vi "haoFPGA.vi"() -> ()   [LabVIEW 2018]
uses:
  <vilib>/Platform/TimedLoop/XDataNode/timing_clust.ctl
  <vilib>/Platform/TimedLoop/XDataNode/nitl_modes.ctl
  <vilib>/Platform/TimedLoop/XDataNode/wakeup.ctl
  <vilib>/rvi/Emulation/niFpgaSctlEmulationGetInTimedLoop.vi
  <vilib>/rvi/Emulation/niFpgaEmulationReportErrorSimple.vi
  <vilib>/rvi/Emulation/niFpgaGetClockAttributes.vi
  <vilib>/rvi/Emulation/niFpgaCriticalErrorInLSC.vi
  <vilib>/rvi/Emulation/niFpgaProcessEmulError.vi
  <vilib>/Platform/TimedLoop/XDataNode/XDataNode.xnode
  <vilib>/Platform/TimedLoop/XDataNode/XDNodeRunTimeDep.lvlib
panel:
  in  "B":bool
  in  "A":bool
  out "C":bool
  in  "stop":bool
  in  "DIR2":bool
  in  "ENA2":bool
  in  "STBY2":bool
  in  "CH2 DC":fxp<+,32,0>
  in  "CH1 DC":fxp<+,32,0>
  in  "STBY1":bool
  in  "ENA1":bool
  in  "DIR1":bool
  # "Motor control"
  # "Channel 1"
  # "Channel 2"
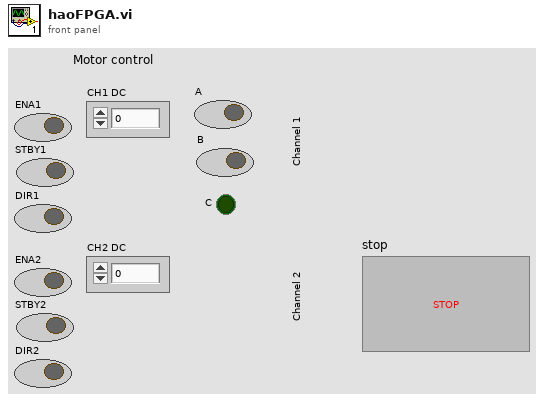
[diagram p1: front panel]
types:
  T1 = cluster{"FPGA I/O":refnum<k21>, "FPGA I/O 2":refnum<k21>, "FPGA I/O 3":refnum<k21>, "FPGA I/O 4":refnum<k21>, "FPGA I/O 5":refnum<k21>, "FPGA I/O 6":refnum<k21>, "FPGA I/O 7":refnum<k21>}
  T2 = typedef "XDNodeRunTimeDep.lvlib/timing_clust.ctl" = cluster{"Expected End [f-1]":u64, "Actual End [f-1]":u64, "Finished Late? [f-1]":bool, "Expected End [i-1]":u64, "Actual End [i-1]":u64, "Finished Late? [i-1]":bool, "Expected Start [i]":u64, "Actual Start [i]":u64, "Expected Start [f]":u64, "Actual Start [f]":u64, "Source Name":string, "Structure Name":string, "Period":i64, "Deadline":i64, "Offset":i64, "Start":i64, "Priority":i32, "Timeout":i32, "Mode":T3, "Wakeup Reason":T4, "Error":errorcluster, "Source Type":string, "Secondary Source Type":string, "Global End Time":u64, "Global Start Time":u64, "Frame Duration":u64, "Iteration Duration":u64, "Assigned CPU":i32, "I/O Scan Engine Mode":u32}
  T3 = typedef "XDNodeRunTimeDep.lvlib/nitl_modes.ctl" = enum32{"No Change", "Process missed periods, maintain original phase", "Discard missed periods, maintain original phase", "Process missed periods, ignore original phase", "Discard missed periods, ignore original phase"}
  T4 = typedef "XDNodeRunTimeDep.lvlib/wakeup.ctl" = enum32{"Normal", "Aborted", "Asynchronous wakeup", "Timing source error", "Timed loop error", "Timeout"}
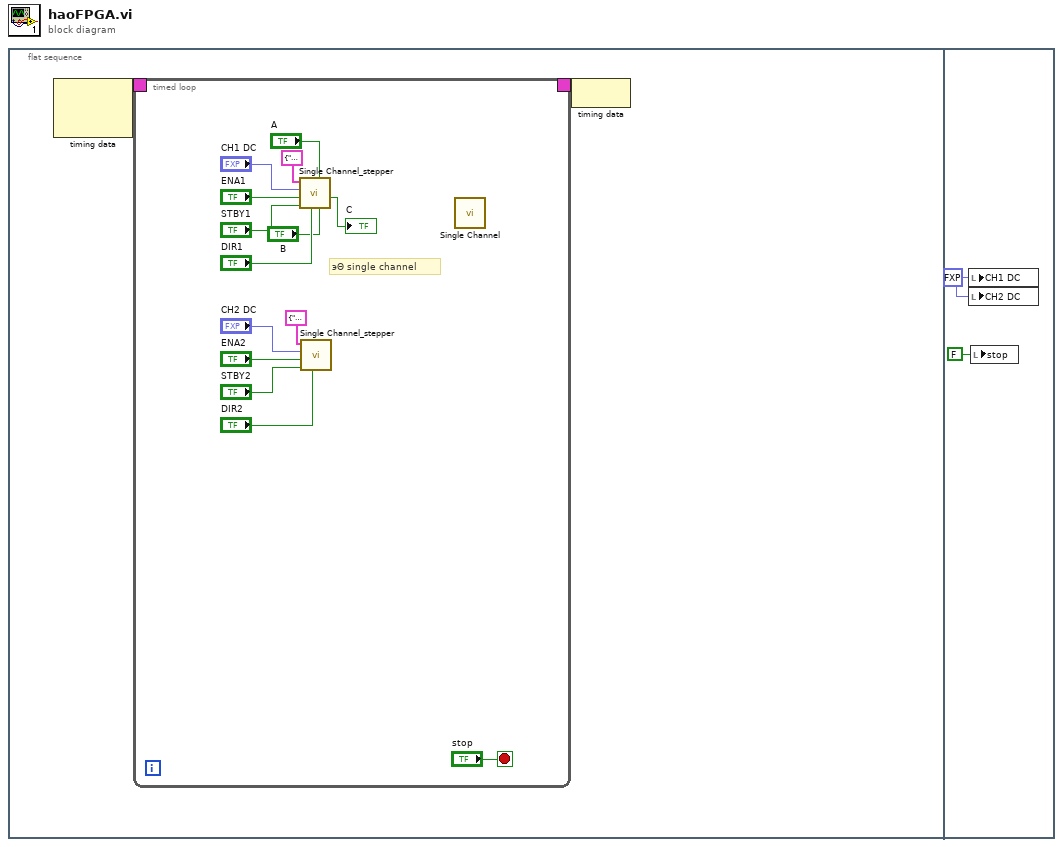
[diagram p0: block diagram]
diagram:
  n1 = flat-sequence {
    frame #0 {
      n2 = node-c288() -> (w2:T2)  [unwired: 2 in]
      n3 = timed-loop {
        timing: w2 -> [_]
        timing-out: [_] -> w1
        stop <- "stop" stop-if-true
        # "эΘ single channel"
        n4 = call "Single Channel_stepper.vi"("B"="B", "A"="A", "DIR"="DIR1", "STBY"="STBY1", "ENA"="ENA1", "Duty"="CH1 DC", "I/O Channel"=T1 {"FPGA I/O"="ConnectorA/DIO6", "FPGA I/O 2"="ConnectorA/DIO5", "FPGA I/O 3"="ConnectorA/DIO4", "FPGA I/O 4"="ConnectorA/DIO3", "FPGA I/O 5"="ConnectorA/DIO2", "FPGA I/O 6"="ConnectorA/DIO1", "FPGA I/O 7"="ConnectorA/DIO0"}) -> ("C"=→"C":bool)  [unwired: 4 in]
        n5 = call "Single Channel_stepper.vi"("DIR"="DIR2", "STBY"="STBY2", "ENA"="ENA2", "Duty"="CH2 DC", "I/O Channel"=T1 {"FPGA I/O"="ConnectorA/DIO13", "FPGA I/O 2"="ConnectorA/DIO12", "FPGA I/O 3"="ConnectorA/DIO11", "FPGA I/O 4"="ConnectorA/DIO10", "FPGA I/O 5"="ConnectorA/DIO9", "FPGA I/O 6"="ConnectorA/DIO8", "FPGA I/O 7"="ConnectorA/DIO7"}) -> ()  [unwired: 6 in, 1 out]
        n6 = call "Single Channel.vi"() -> ()  [unwired: 9 in, 3 out]
      }
      n7 = node-c288(w1) -> ()
    }
    frame #1 {
      w22 = fxp<+,32,0> 0.0 ("CH1 DC")
      n8 = local write "CH1 DC"(w22) -> ()
      n9 = local write "CH2 DC"(w22) -> ()
      n10 = local write "stop"(FALSE ("stop")) -> ()
    }
  }
